vi "Word Find Application Directory.vi"(11 "error in":errorcluster) -> (4 "application directory":path, 15 "error out":errorcluster)   [LabVIEW 2017, in "NI_ReportGenerationToolkit.lvlib"]
uses:
  <vilib>/addons/_office/NI_ReportGenerationToolkit.lvlib
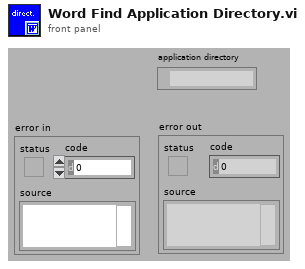
[diagram p1: front panel]
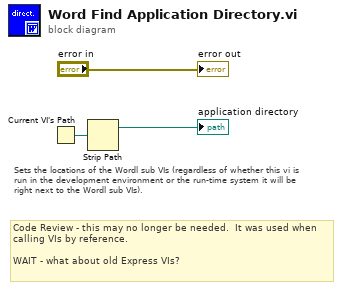
[diagram p0: block diagram]
diagram:
  # "Code Review - this may no longer be needed.  It was used when calling VIs by reference.\n\nWAIT - what about old Express VIs?"
  # "Sets the locations of the Wordl sub VIs (regardless of whether this vi is run in the development environment or the run-time system it will be right next to the Wordl sub VIs)."
  n1 = Current VI's Path() -> (path=w1:path)
  n2 = Strip Path(path=w1) -> (stripped path=→"application directory":path)  [unwired: 1 out]
  "error out" <- "error in"
